vi "Load_Profile.vi"(1 "Offset":dbl, 2 "Frequency":dbl, 3 "Amplitude":dbl, 4 "Loop Index":dbl) -> (0 "Load Index":dbl)   [LabVIEW 2018]
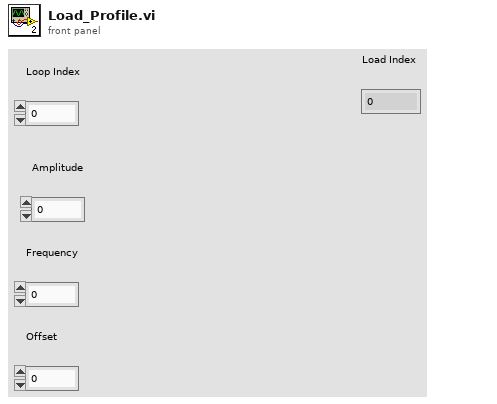
[diagram p1: front panel]
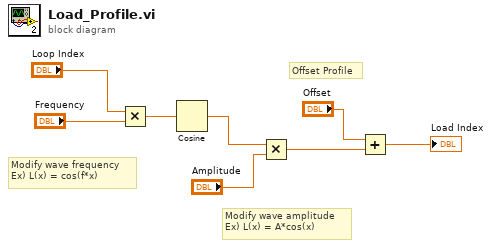
[diagram p0: block diagram]
diagram:
  # "Offset Profile"
  # "Modify wave frequency\nEx) L(x) = cos(f*x)"
  # "Modify wave amplitude\nEx) L(x) = A*cos(x)"
  n1 = Multiply(x="Loop Index", y="Frequency") -> (x*y=w4:dbl)
  n2 = Cosine(x=w4) -> (cos(x)=w8:dbl)
  n3 = Multiply(x=w8, y="Amplitude") -> (x*y=w2:dbl)
  n4 = Add(x="Offset", y=w2) -> (x+y=→"Load Index":dbl)
